vi "save configuration.vi"(10 "Waveform chart":refnum<vi>, 11 "selected parameters":string[](array[string])) -> ()   [LabVIEW 2016]
uses:
  configuration file type def.ctl
  Communication Global variables.vi
  <vilib>/addons/_JKI.lib/Serialization/JSON/JKI JSON Serialization.lvlib
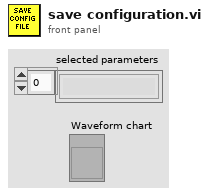
[diagram p1: front panel]
types:
  T1 = typedef "configuration file type def.ctl" = cluster{"selected parameters":string[], "REST URL":string, "UDP port":u16, "XScale.Minimum":dbl, "XScale.Maximum":dbl, "Yscale mins":dbl[], "Yscale maxs":dbl[], "Yscale colors":u32[], "LegNumRows":u32, "plot colors":u32[], "plot pointstyles":u8[], "plot names":string[], "plot yscale selections":u32[], "plot visibles":bool[]}
  T2 = enum16{"open", "replace", "create", "open or create", "replace or create", "replace or create with confirmation"}
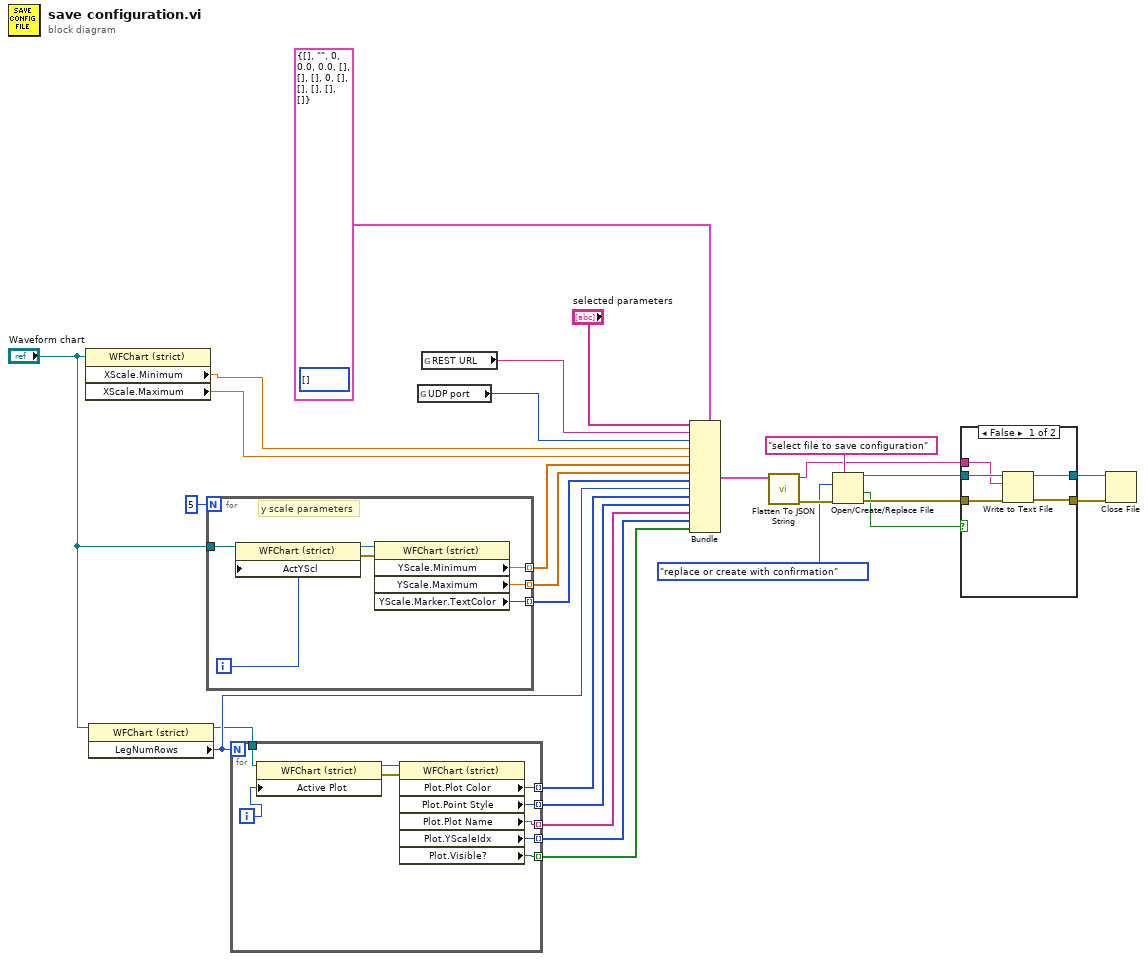
[diagram p0: block diagram]
diagram:
  (unwired) i32[] []
  n1 = property class="WFChart (strict)"(reference="Waveform chart") -> ("XScale.Minimum"=w25:dbl, "XScale.Maximum"=w24:dbl)  [unwired: 1 in, 2 out]
  n2 = property class="WFChart (strict)"(reference="Waveform chart") -> (reference out=w8:refnum<vi>, "LegNumRows"=w19:u32)  [unwired: 1 in, 1 out]
  n3 = for {
    N: 5 -> [_]
    tunnel: "Waveform chart" -> [w34]
    tunnel: [w31] -> w23 mode=indexing
    tunnel: [w30] -> w22 mode=indexing
    tunnel: [w29] -> w21 mode=indexing
    i -> [w35]
    # "y scale parameters"
    n4 = property class="WFChart (strict)"(reference=w34, "ActYScl"=w35) -> (reference out=w33:refnum<vi>, error out=w32:errorcluster)  [unwired: 1 in]
    n5 = property class="WFChart (strict)"(reference=w33, error in=w32) -> ("YScale.Minimum"=w31:dbl, "YScale.Maximum"=w30:dbl, "YScale.Marker.TextColor"=w29:u32)  [unwired: 2 out]
  }
  n6 = for {
    N: w19 -> [_]
    tunnel: [w41] -> w18 mode=indexing
    tunnel: [w40] -> w17 mode=indexing
    tunnel: [w39] -> w16 mode=indexing
    tunnel: [w38] -> w15 mode=indexing
    tunnel: [w37] -> w14 mode=indexing
    tunnel: w8 -> [w36]
    i -> [w44]
    n7 = property class="WFChart (strict)"(reference=w36, "Active Plot"=w44) -> (reference out=w42:refnum<vi>, error out=w43:errorcluster)  [unwired: 1 in]
    n8 = property class="WFChart (strict)"(reference=w42, error in=w43) -> ("Plot.Plot Color"=w41:u32, "Plot.Point Style"=w40:u8, "Plot.Plot Name"=w39:string, "Plot.YScaleIdx"=w38:u32, "Plot.Visible?"=w37:bool)  [unwired: 2 out]
  }
  n9 = global read "Communication Global variables.vi" "UDP port"() -> (w5:u16)
  n10 = global read "Communication Global variables.vi" "REST URL"() -> (w6:string)
  n11 = Bundle(cluster=T1 {"selected parameters"=[], "REST URL"="", "UDP port"=0, "XScale.Minimum"=0.0, "XScale.Maximum"=0.0, "Yscale mins"=[], "Yscale maxs"=[], "Yscale colors"=[], "LegNumRows"=0, "plot colors"=[], "plot pointstyles"=[], "plot names"=[], "plot yscale selections"=[], "plot visibles"=[]} ("output cluster"), "selected parameters"="selected parameters", "REST URL"=w6, "UDP port"=w5, "XScale.Minimum"=w25, "XScale.Maximum"=w24, "Yscale mins"=w23, "Yscale maxs"=w22, "Yscale colors"=w21, "LegNumRows"=w19, "plot colors"=w18, "plot pointstyles"=w17, "plot names"=w16, "plot yscale selections"=w15, "plot visibles"=w14) -> (w13:T1)
  n12 = call <vilib>:"Flatten To JSON String.vi"("Variant"=w13) -> ("error out"=w12:errorcluster, "JSON String"=w9:string)  [unwired: 9 in]
  n13 = Open/Create/Replace File(error in=w12, prompt="select file to save configuration", operation (0:open)=T2."replace or create with confirmation") -> (refnum out=w10:refnum<file>, cancelled=w3:bool, error out=w11:errorcluster)  [unwired: 3 in]
  n14 = case shown="False" w3 {
    tunnel: w11 -> [w49 w50]
    tunnel: w10 -> [w48 w51]
    tunnel: w9 -> [w47 _]
    tunnel: [w46 w51] -> w2
    tunnel: [w45 w50] -> w1
    frame False {
      n15 = Write to Text File(file (use dialog)=w48, text=w47, error in=w49) -> (refnum out=w46:refnum<file>, error out=w45:errorcluster)  [unwired: 1 in, 1 out]
    }
    frame True {
    }
  }
  n16 = Close File(refnum=w2, error in=w1) -> ()  [unwired: 2 out]
